vi "GetDaysCount.vi"(10 "month":string, 11 "year":string) -> (3 "Numeric":i32)   [LabVIEW 2017, in "UI_TimeSelector.xctl"]
uses:
  UI_TimeSelector.xctl
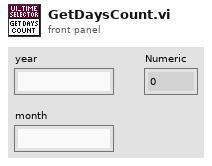
[diagram p1: front panel]
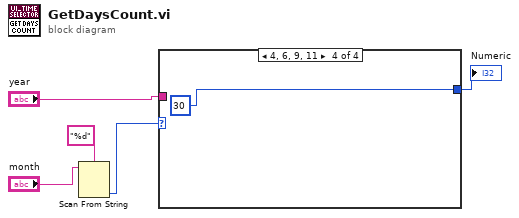
[diagram p0: block diagram]
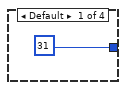
[diagram p2: hidden frame]
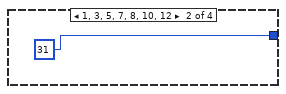
[diagram p3: hidden frame]
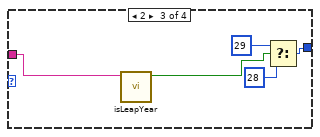
[diagram p4: hidden frame]
diagram:
  n1 = Scan From String(format string="%d", input string="month") -> (output 1=w3:i32)  [unwired: 3 in, 3 out]
  n2 = case shown="4, 6, 9, 11" w3 {
    tunnel: [31 31 w8 30] -> w2
    tunnel: "year" -> [_ _ w12 _]
    frame Default {
    }
    frame 1, 3, 5, 7, 8, 10, 12 {
    }
    frame 2 {
      n3 = call "isLeapYear.vi"("year"=w12) -> ("Boolean"=w9:bool)  [unwired: 10 in]
      n4 = Select(t=29, s=w9, f=28) -> (s? t:f=w8:i32)
    }
    frame 4, 6, 9, 11 {
    }
  }
  "Numeric" <- w2
